vi "稱號-神準無比.vi"() -> ()   [LabVIEW 2014]
panel:
  in  "退出視窗":bool
  # "恭喜獲得稱號:"
  # "能猜中那麼多次，你是不是有超能力可以去看到\n骰盅內的點數啊~"
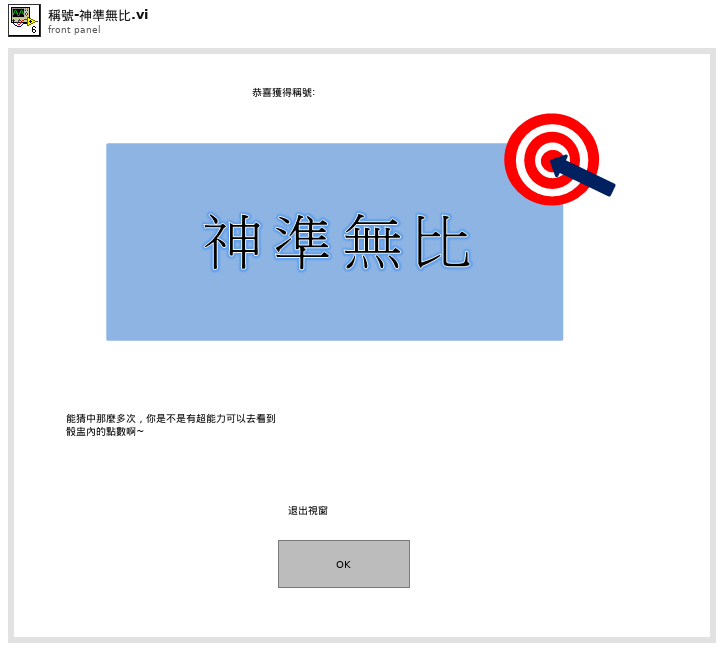
[diagram p1: front panel]
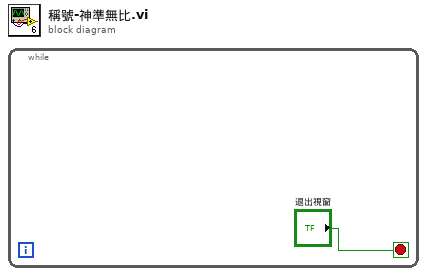
[diagram p0: block diagram]
diagram:
  n1 = while {
    stop <- "退出視窗" stop-if-true
  }
